vi "D-HParameters.vi"(2 "n+1":T1, 3 "Start":T2=[[1.0, 0.0, 0.0, 0.0], [0.0, 1.0, 0.0, 0.0], [0.0, 0.0, 1.0, 0.0], [0.0, 0.0, 0.0, 1.0]]) -> (1 "A x B":T2)   [LabVIEW 2024]
uses:
  <vilib>/Analysis/Matrix/Datatypes/RealMatrix.ctl
  <vilib>/Analysis/baseanly.llb/Real A x B.vi
  <vilib>/Analysis/NI_AALBase.lvlib
  <vilib>/Analysis/Matrix/NI_Matrix.lvlib
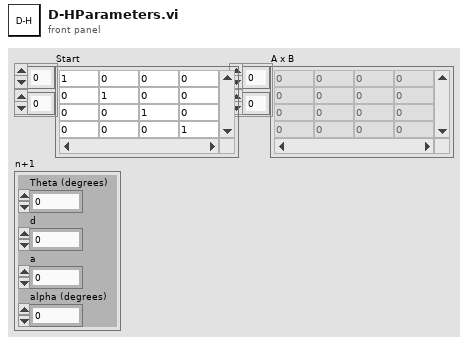
[diagram p1: front panel]
types:
  T1 = cluster{"Theta (degrees)":dbl, "d":dbl, "a":dbl, "alpha (degrees)":dbl}
  T2 = typedef "NI_Matrix.lvlib/RealMatrix.ctl" = dbl[][]
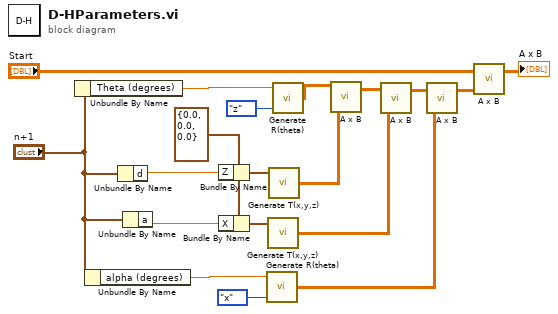
[diagram p0: block diagram]
diagram:
  w2 = cluster{"X":dbl, "Y":dbl, "Z":dbl} {"X"=0.0, "Y"=0.0, "Z"=0.0} ("Translation")
  n1 = Unbundle By Name("n+1") -> ("Theta (degrees)"=w6:dbl)
  n2 = Unbundle By Name("n+1") -> ("alpha (degrees)"=w9:dbl)
  n3 = Unbundle By Name("n+1") -> ("d"=w1:dbl)
  n4 = Unbundle By Name("n+1") -> ("a"=w3:dbl)
  n5 = Bundle By Name(cluster=w2, "Z"=w1) -> (w7:cluster{"X":dbl, "Y":dbl, "Z":dbl})
  n6 = Bundle By Name(cluster=w2, "X"=w3) -> (w8:cluster{"X":dbl, "Y":dbl, "Z":dbl})
  n7 = call <userlib>:"Generate R(theta).vi"("Axis"=enum16{"x", "y", "z"}."x", "Angle (degrees)"=w9) -> ("Transformation Matrix"=w16:T2)  [unwired: 1 in]
  n8 = call <userlib>:"Generate T(x,y,z).vi"("Translation"=w8) -> ("Transformation Matrix"=w14:T2)  [unwired: 2 in]
  n9 = call <userlib>:"Generate T(x,y,z).vi"("Translation"=w7) -> ("Transformation Matrix"=w12:T2)  [unwired: 2 in]
  n10 = call <userlib>:"Generate R(theta).vi"("Axis"=enum16{"x", "y", "z"}."z", "Angle (degrees)"=w6) -> ("Transformation Matrix"=w11:T2)  [unwired: 1 in]
  n11 = call-poly <vilib>:"A x B.vi"("B"=w12, "A"=w11) -> ("A x B"=w13:T2)  [unwired: 1 out]
  n12 = call-poly <vilib>:"A x B.vi"("B"=w14, "A"=w13) -> ("A x B"=w15:T2)  [unwired: 1 out]
  n13 = call-poly <vilib>:"A x B.vi"("B"=w16, "A"=w15) -> ("A x B"=w17:T2)  [unwired: 1 out]
  n14 = call-poly <vilib>:"A x B.vi"("B"=w17, "A"="Start") -> ("A x B"=→"A x B":T2)  [unwired: 1 out]
